vi "Load Configuration.vi"(0 "INI Configuration in":refnum<class "TLB` Configuration.lvclass">, 5 "INI file path in":path, 11 "error in (no error)":errorcluster) -> (4 "INI Configuration out":refnum<class "TLB` Configuration.lvclass">, 15 "error out":errorcluster)   [LabVIEW 2026, in "Synchronize AWS S3 Content.lvlib" / "TLB` Configuration.lvclass"]
uses:
  TLB` Configuration.lvclass
  TLB` Configuration.lvclass/TLB` Configuration.ctl
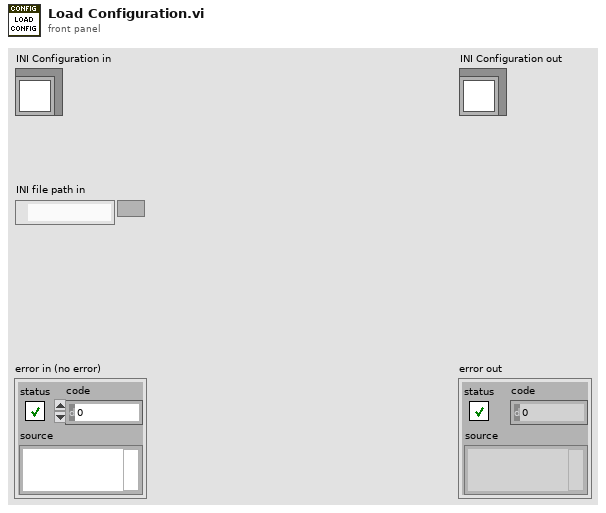
[diagram p1: front panel]
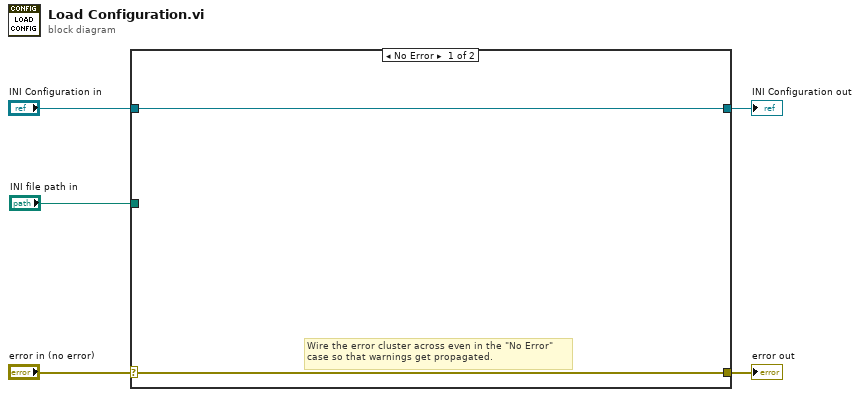
[diagram p0: block diagram]
diagram:
  n1 = case shown="No Error" "error in (no error)" {
    selector: "error in (no error)" -> [w6 w9]
    tunnel: [w6 w9] -> w4
    tunnel: [w7 w8] -> w2
    tunnel: "INI Configuration in" -> [w7 w8]
    tunnel: "INI file path in" -> [_ _]
    frame No Error {
      # "Wire the error cluster across even in the \"No Error\"\ncase so that warnings get propagated."
    }
    frame Error {
    }
  }
  "error out" <- w4
  "INI Configuration out" <- w2
